vi "Main.vi"(11 "Module Admin":refnum<class "Delacor_lib_QMH_Module Admin.lvclass">) -> ()   [LabVIEW 2022 SP3, in "ActorModule.lvlib"]
doc: "This template is based off of the Queued Message Handler design pattern and the Queued Message Handler project template that ships with LabVIEW.\n\nThe main difference is that the queue is private to this module and communication between modules is performed via Broadcast and Request events.\n\nRequest events are wrapped in public API methods and are handled in the Event Handling Loop (EHL) of this VI. Any module can register for Broadcast events sent by this module. The EHL generates messages based on user interface actions.\n\nThe Message Handling Loop (MHL) processes messages generated by the EHL, or by other messages. The messages are string values, so new messages can be added easily to the Message Cases case structure in the MHL. Each message cluster can also provide an optional value for Message Data, which is a variant that can be converted to whatever message-specific data is required.\n____\nHAMPEL SOFTWARE ENGINEERING v2.6.0 (2023-12-19 10:54)"
uses:
  ActorModule.lvlib
  <vilib>/Delacor/Delacor QMH/Libraries/Module Admin_class/Delacor_lib_QMH_Module Admin.lvclass
  Libraries/hse-libraries/Source/hse-dqmh/Controls/System Message Source.ctl
  Framework/UI Manager/System Message Argument--cluster.ctl
  Module Data--cluster.ctl
  Stop Argument--cluster.ctl
  <vilib>/Delacor/Delacor QMH/Libraries/Message Queue_class/Delacor_lib_QMH_Message Queue.lvclass/Delacor_lib_QMH_Message Queue.ctl
  <vilib>/Delacor/Delacor QMH/Libraries/Module Admin_class/Delacor_lib_QMH_Module Admin.lvclass/Delacor_lib_QMH_Module Admin.ctl
  Prepare Argument--cluster.ctl
  Configure Argument--cluster.ctl
  Request UI Display Argument--cluster.ctl
  Libraries/hse-libraries/Source/hse-dqmh/Controls/Module Display Scenarios.ctl
  Request UI Display (Reply Payload)--cluster.ctl
  Framework/Navigation/Sub-VIs/Ctl Target.ctl
  <vilib>/Utility/miscctls.llb/LVPointTypeDef.ctl
  <vilib>/Delacor/Delacor QMH/Libraries/Message Queue_class/Delacor_lib_QMH_Enqueue Message (Single).vi
  <vilib>/Delacor/Delacor QMH/Libraries/Module Admin_class/Delacor_lib_QMH_Get External Launch.vi
  <vilib>/Utility/error.llb/Error Cluster From Error Code.vi
  <vilib>/ErrorRing/Error Ring.xnode
  <vilib>/Delacor/Delacor QMH/Libraries/Message Queue_class/Delacor_lib_QMH_Message Queue.lvclass
  Libraries/hse-libraries/Source/hse-configuration/config-ini/config-ini.lvclass
  Framework/UI Manager/UI Manager.lvlib
  Libraries/hse-libraries/Source/hse-dqmh/hse-dqmh.lvlib
  <vilib>/Hampel Software Engineering/HSE Logger/hse-logger.lvlib
  Framework/Navigation/Navigation.lvlib
panel:
  out "Message Time":timestamp
  out "Payload":variant
  out "Source":T1
  out "Identifier":string
  in  "Timeout [ms]":u32
  out "Timeout Counter":u32
  out "error out":errorcluster
  # "The \"ActorModule\" serves as an example of a module with a helper loop, which comes with two features: \n\n1. The helper loop can be \"enabled\" to run continuously by using the timeout case of its event structure. It \nwill then increase the timeout counter shown in the indicator below, and it will rotate the selection inside \nthe listbox which is shown in the navigation menu to the left when selecting the \"Actor Module\" button. \n\n2. The helper loop can be registered to receive external events, i.e. broadcasts from other DQMH modules. \nWhen registered for the UI Manager's broadcast event, the indicators below will show any System Message \nthe UI Manager broadcasts, for example whenever a module is removed from the UI Managers subpanel.\n\nThe helper loop can be operated by pressing the \"Actor Module Actions\" button in the navigation menu to \nthe left and then selecting items from the listbox that appears below the button."
  # "Helper Loop - Timeout"
  # "Helper Loop - Broadcast Registration"
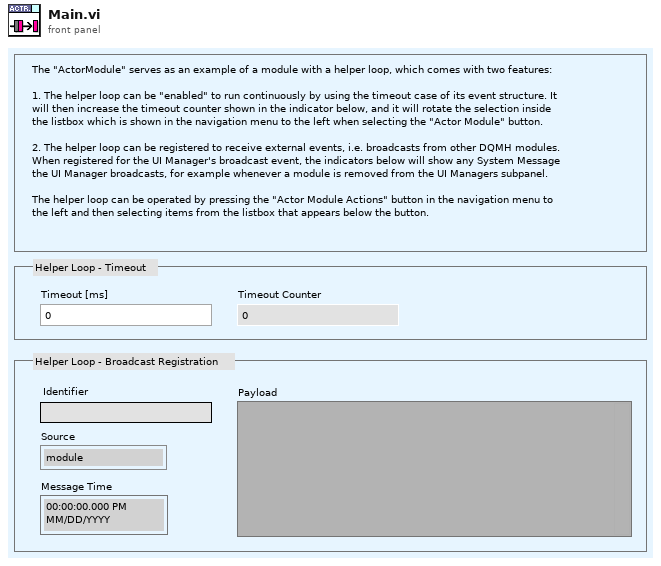
[diagram p1: front panel]
types:
  T1 = typedef "hse-dqmh.lvlib/System Message Source.ctl" = enum16{"module", "application", "network"}
  T2 = typedef "Navigation.lvlib/Broadcast Events--cluster.ctl" = cluster{"Module Did Init":refnum<user-event>, "Status Updated":refnum<user-event>, "Error Reported":refnum<user-event>, "Module Did Stop":refnum<user-event>, "Update Module Execution Status":refnum<user-event>, "Button Pressed":refnum<user-event>, "Sub-Control Pressed":refnum<user-event>, "System Message":refnum<user-event>}
  T3 = typedef "ActorModule.lvlib/Request Events--cluster.ctl" = cluster{"Stop Module":refnum<user-event>, "Show Panel":refnum<user-event>, "Hide Panel":refnum<user-event>, "Get Module Execution Status":refnum<user-event>, "Show Diagram":refnum<user-event>, "Prepare":refnum<user-event>, "Configure":refnum<user-event>, "Enable Actor":refnum<user-event>, "Disable Actor":refnum<user-event>, "Register for System Messages":refnum<user-event>, "Unregister from System Messages":refnum<user-event>, "Request UI Display":refnum<user-event>}
  T4 = typedef "ActorModule.lvlib/Module Data--cluster.ctl" = cluster{"Status":string, "WES Raw Data":cluster{"pdoX":waveform(dbl), "pdoZ":waveform(dbl)}}
  T5 = typedef "Navigation.lvlib/Ctl Target.ctl" = enum16{"Top Button", "Sub ListBox"}
  T6 = enum32{"invalid lock state", "Not Locked", "Locked (No Password)", "Password-protected"}
  T7 = typedef "ActorModule.lvlib/Stop Argument--cluster.ctl" = cluster{"Origin":string, "Exit via Stop Module Req?":bool, "Wait for Module to stop?":bool}
  T8 = typedef "ActorModule.lvlib/Prepare Argument--cluster.ctl" = cluster{"Boolean":bool}
  T9 = typedef "ActorModule.lvlib/Configure Argument--cluster.ctl" = cluster{"Boolean":bool}
  T10 = typedef "ActorModule.lvlib/Request UI Display Argument--cluster.ctl" = cluster{"Scenario":T11, "Wait Notifier":refnum<notifier>, "wait for reply":bool}
  T11 = typedef "hse-dqmh.lvlib/Module Display Scenarios.ctl" = enum16{"Stand-Alone", "Managed"}
  T12 = typedef "LVPointTypeDef.ctl" = cluster{"Horizontal":i16, "Vertical":i16}
  T13 = enum32{"Invalid", "Standard", "Closed", "Hidden", "Minimized", "Maximized"}
  T14 = typedef "ActorModule.lvlib/Request UI Display (Reply Payload)--cluster.ctl" = cluster{"Accept?":bool, "error":errorcluster}
  T15 = typedef "eventsource.ctl" = u32
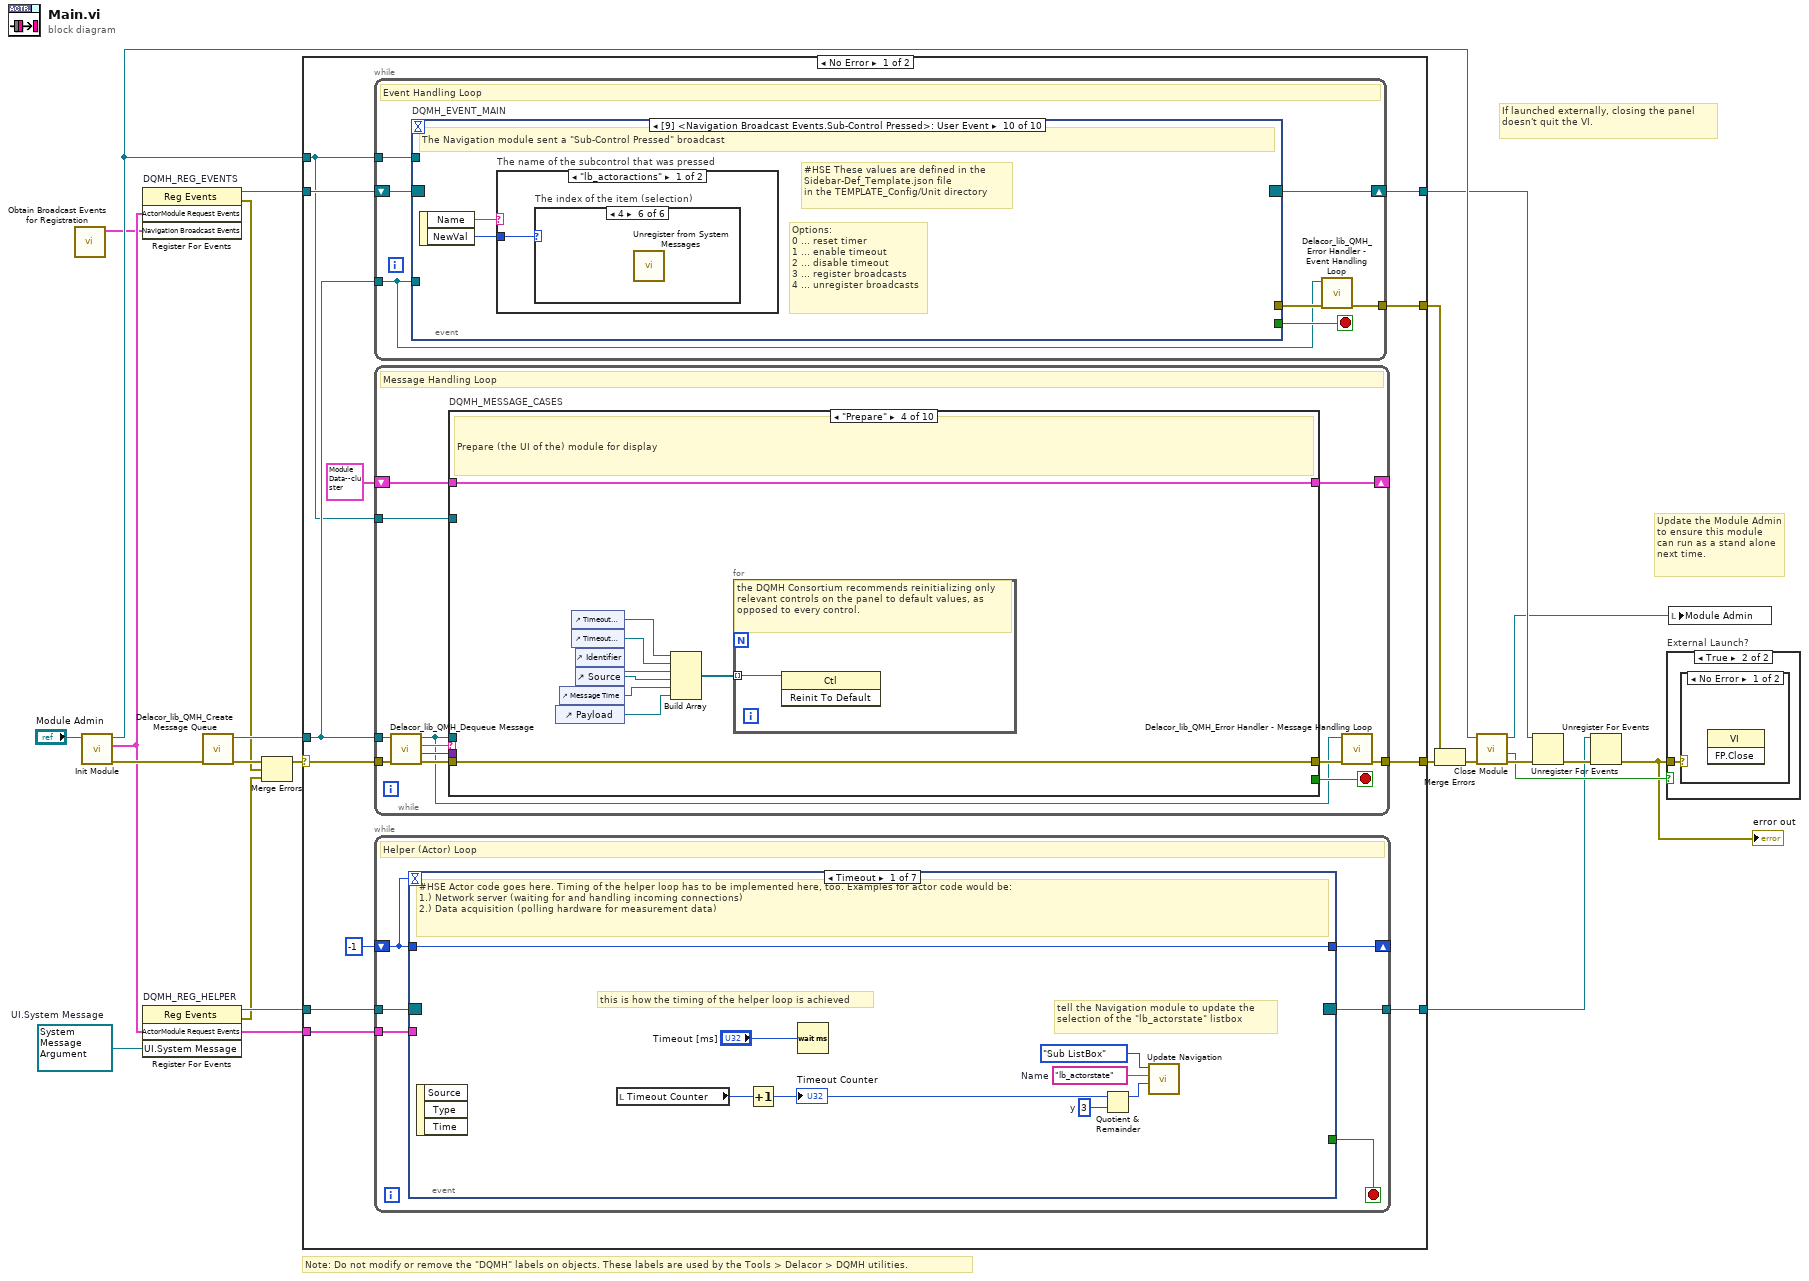
[diagram p0: block diagram]
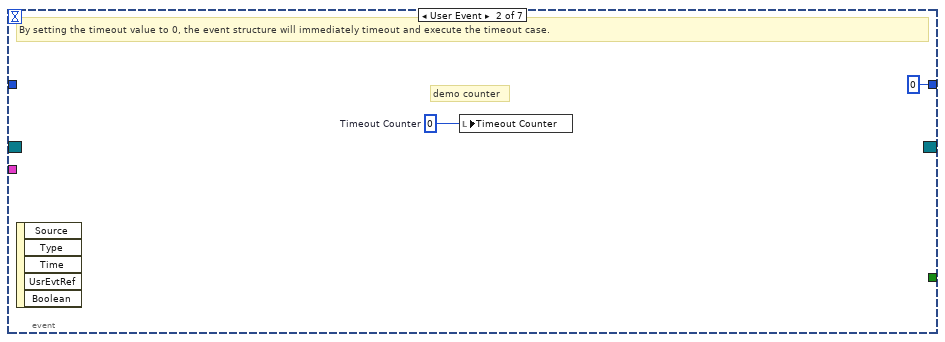
[diagram p2: hidden frame]
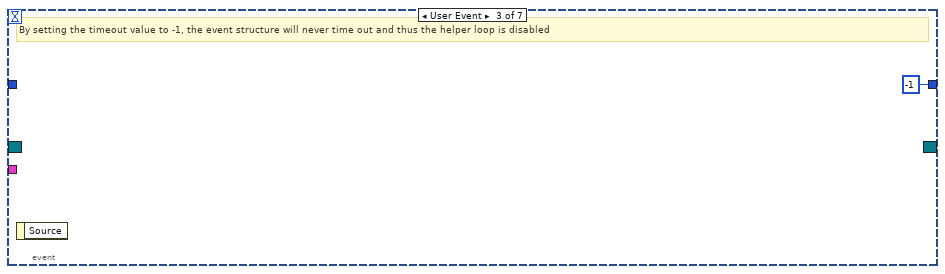
[diagram p3: hidden frame]
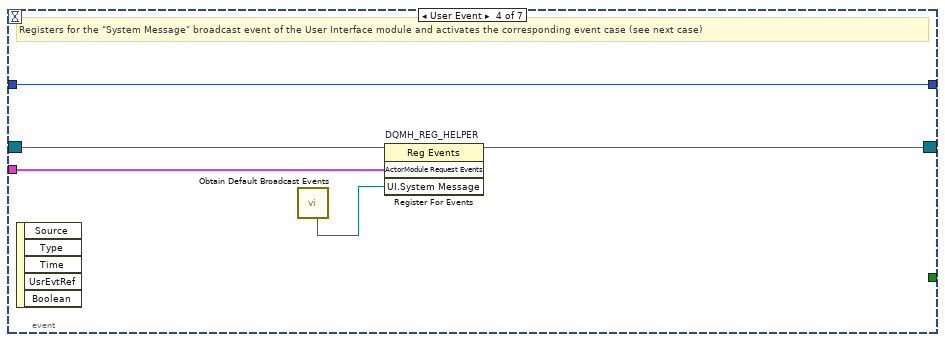
[diagram p4: hidden frame]
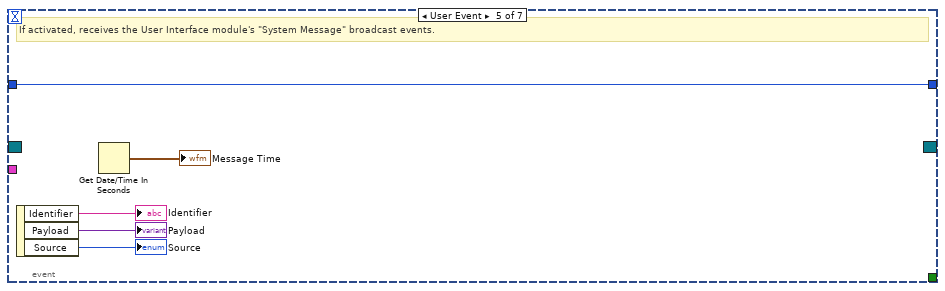
[diagram p5: hidden frame]
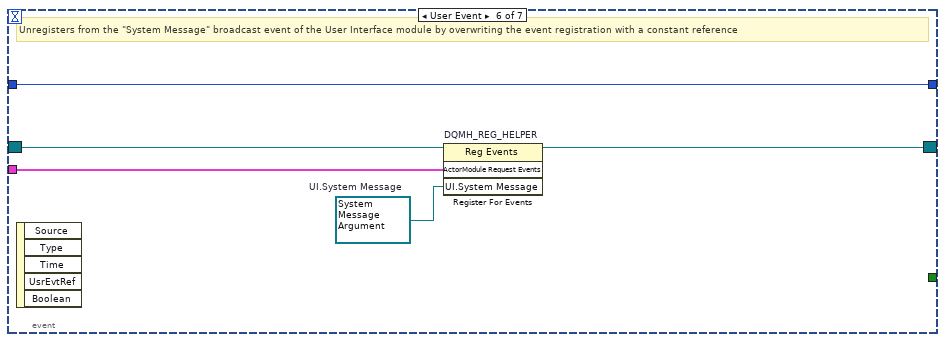
[diagram p6: hidden frame]
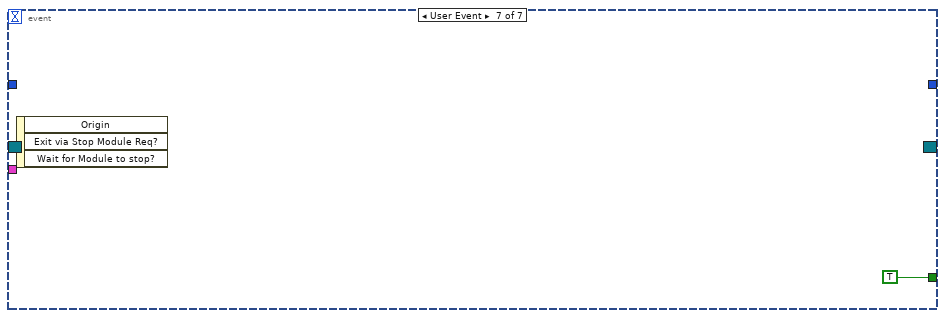
[diagram p7: hidden frame]
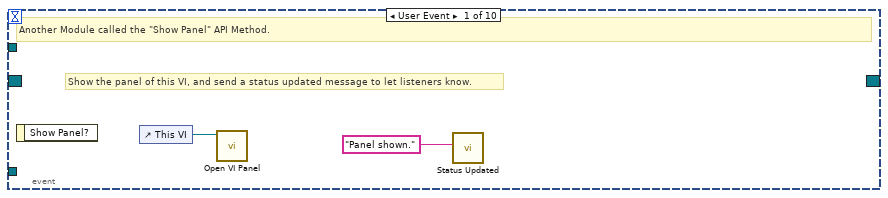
[diagram p8: hidden frame]
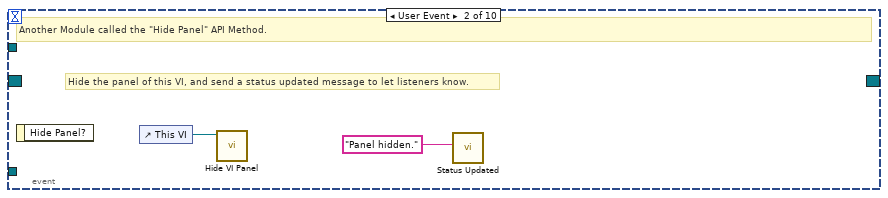
[diagram p9: hidden frame]
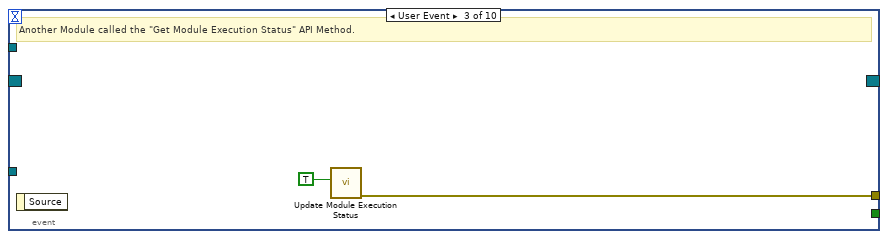
[diagram p10: hidden frame]
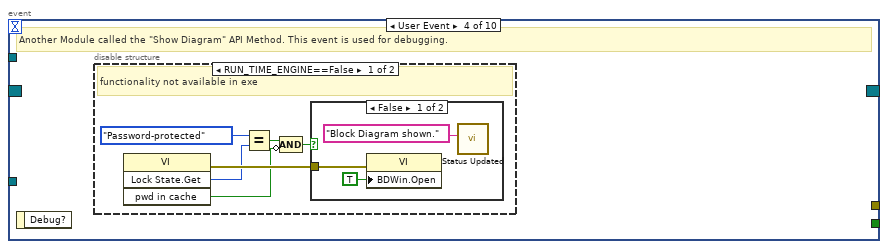
[diagram p11: hidden frame]
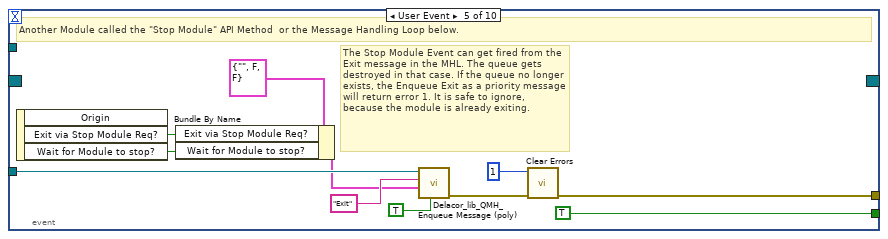
[diagram p14: hidden frame]
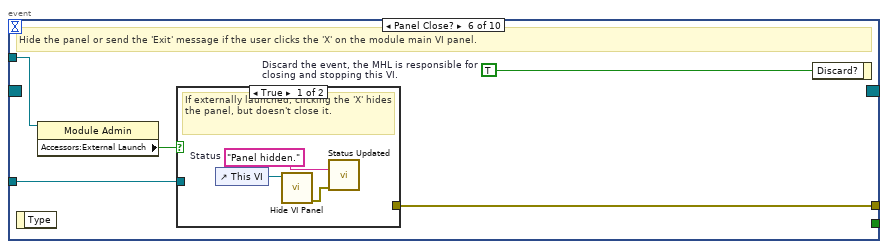
[diagram p15: hidden frame]
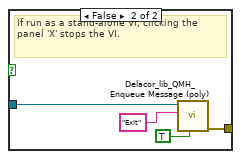
[diagram p16: hidden frame]
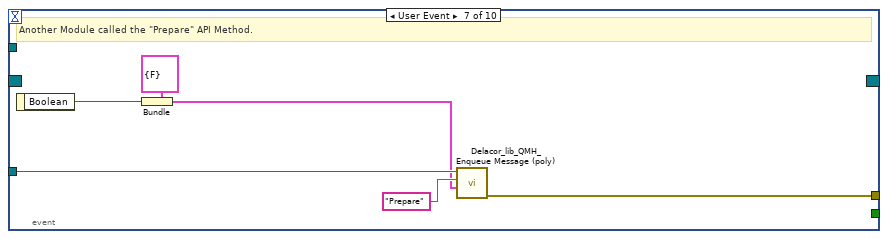
[diagram p17: hidden frame]
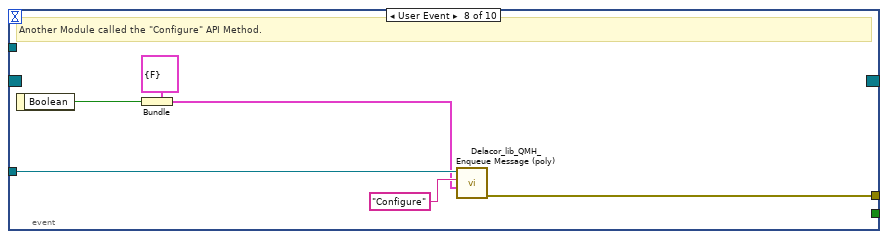
[diagram p18: hidden frame]
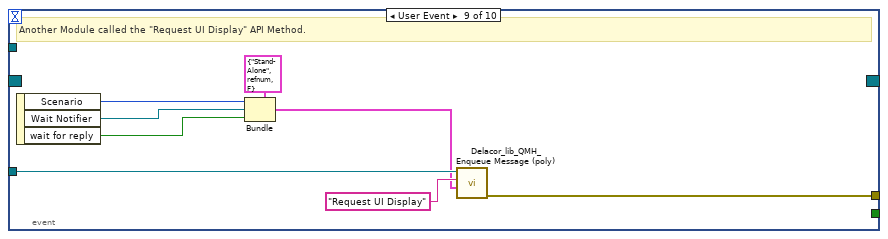
[diagram p19: hidden frame]
diagram:
  w6 = refnum<user-event> refnum  # UI.System Message
  # "If launched externally, closing the panel doesn't quit the VI."
  # "Note: Do not modify or remove the \"DQMH\" labels on objects. These labels are used by the Tools > Delacor > DQMH utilities."
  # "Update the Module Admin to ensure this module can run as a stand alone next time."
  n1 = call "Obtain Broadcast Events for Registration.vi"() -> ("Navigation Broadcast Events"=w1:T2)  [unwired: 9 in, 2 out]
  n2 = call "Init Module.vi"("Singleton Module Admin in"="Module Admin") -> ("error out"=w21:errorcluster, "ActorModule Request Events"=w5:T3, "Singleton Module Admin out"=w23:refnum<class "Delacor_lib_QMH_Module Admin.lvclass">)  [unwired: 8 in]
  n3 = register-events "DQMH_REG_EVENTS"(w5, w1) -> (reference out=w19:refnum<event-registration>, error out=w9:errorcluster)  [unwired: 2 in]
  n4 = register-events "DQMH_REG_HELPER"(w5, w6) -> (reference out=w8:refnum<event-registration>, error out=w7:errorcluster)  [unwired: 2 in]
  n5 = call <vilib>:"Delacor_lib_QMH_Create Message Queue.vi"("error in"=w21) -> ("error out"=w11:errorcluster, "Message Queue"=w18:refnum<class "Delacor_lib_QMH_Message Queue.lvclass">)  [unwired: 9 in]
  n6 = Merge Errors(w11, w9, w7) -> (w10:errorcluster)
  n7 = case shown="No Error" w10 {
    selector: w10 -> [w29 w277]
    tunnel: [w35 w277] -> w22
    tunnel: [w34 w282] -> w20
    tunnel: w19 -> [w32 w282]
    tunnel: w18 -> [w31 w273]
    tunnel: [w30 _] -> w14
    tunnel: w23 -> [w28 w278]
    tunnel: w8 -> [w27 w274]
    tunnel: w5 -> [w25 _]
    tunnel: [w24 w274] -> w2
    frame No Error {
      n8 = while {
        tunnel: w31 -> [w69]
        shift-right: [w74] -> w34
        shift-left: w32 -> [w75]
        tunnel: [w71] -> w30
        tunnel: w28 -> [w70]
        stop <- w72 stop-if-true
        # "Event Handling Loop"
        n9 = event "DQMH_EVENT_MAIN" shown="[9] <Navigation Broadcast Events.Sub-Control Pressed>: User Event" {
          selector: w75 -> [_ _ _ _ _ _ _ _ _ _]
          dyn-events: [_ _ _ _ _ _ _ _ _ _] -> w74
          timeout: _ -> [_ _ _ _ _ _ _ _ _ _]
          tunnel: [_ _ _ _ TRUE ("Discard?") _ _ _ _ _] -> w72
          tunnel: w69 -> [_ _ _ _ w99 w105 w119 w125 w133 _]
          tunnel: [_ _ w81 _ w95 w104 w114 w120 w129 _] -> w73
          tunnel: w70 -> [_ _ _ _ _ w103 _ _ _ _]
          event User Event {
            # "Show the panel of this VI, and send a status updated message to let listeners know."
            # "Another Module called the \"Show Panel\" API Method."
            n10 = event-data() -> ()  [unwired: 1 in, 1 out]
            n11 = control-ref of="This VI"() -> (w77:refnum<vi>)
            n12 = call "Open VI Panel.vi"("VI"=w77) -> ()  [unwired: 10 in, 1 out]
            n13 = call "Status Updated.vi"("Status"="Panel shown." ("format string")) -> ()  [unwired: 10 in, 1 out]
          }
          event User Event {
            # "Hide the panel of this VI, and send a status updated message to let listeners know."
            # "Another Module called the \"Hide Panel\" API Method."
            n14 = event-data() -> ()  [unwired: 1 in, 1 out]
            n15 = control-ref of="This VI"() -> (w79:refnum<vi>)
            n16 = call "Hide VI Panel.vi"("VI"=w79) -> ()  [unwired: 10 in, 1 out]
            n17 = call "Status Updated.vi"("Status"="Panel hidden." ("format string")) -> ()  [unwired: 10 in, 1 out]
          }
          event User Event {
            # "Another Module called the \"Get Module Execution Status\" API Method."
            n18 = event-data() -> ()  [unwired: 1 in, 1 out]
            n19 = call "Update Module Execution Status.vi"("Running?"=TRUE) -> ("error out"=w81:errorcluster)  [unwired: 10 in]
          }
          event User Event {
            # "Another Module called the \"Show Diagram\" API Method. This event is used for debugging."
            n20 = event-data() -> ()  [unwired: 1 in, 1 out]
            n21 = disable-structure shown="RUN_TIME_ENGINE==False" {
              frame condition #0 (active) {
                # "functionality not available in exe"
                n22 = invoke class="VI" method="Lock State.Get"() -> (error out=w87:errorcluster, "Get Lock State"=w86:T6, "pwd in cache"=w83:bool)  [unwired: 4 in, 1 out]
                n23 = Equal?(x=T6."Password-protected", y=w86) -> (x = y?=w84:bool)
                n24 = Compound Arithmetic op=AND(w84, invert w83) -> (w82:bool)
                n25 = case shown="False" w82 {
                  tunnel: w87 -> [w88 _]
                  frame False {
                    n26 = property class="VI"(error in=w88, "BDWin.Open"=TRUE ("Block Diagram Window:Open")) -> ()  [unwired: 1 in, 2 out]
                    n27 = call "Status Updated.vi"("Status"="Block Diagram shown." ("format string")) -> ()  [unwired: 10 in, 1 out]
                  }
                  frame True {
                    # "Password-protected VI, and the password is not in the cache. Do not show the diagram."
                  }
                }
              }
              frame condition #1 {
              }
            }
          }
          event User Event {
            # "The Stop Module Event can get fired from the Exit message in the MHL. The queue gets destroyed in that case. If the queue no longer exists, the Enqueue Exit as a priority message will return error 1. It is safe to ignore, because the module is already exiting."
            # "Another Module called the \"Stop Module\" API Method  or the Message Handling Loop below."
            n28 = event-data() -> ("Exit via Stop Module Req?"=w93:bool, "Wait for Module to stop?"=w92:bool)  [unwired: 1 in, 1 out]
            n29 = Bundle By Name(cluster=T7 {"Origin"="", "Exit via Stop Module Req?"=FALSE, "Wait for Module to stop?"=FALSE} ("Stop Argument"), "Exit via Stop Module Req?"=w93, "Wait for Module to stop?"=w92) -> (w91:T7)
            n30 = call-poly <vilib>:"Delacor_lib_QMH_Enqueue Message (poly).vi"("Priority Message? (F)"=TRUE, "Message Data"=w91, "Message"="Exit", "Message Queue in"=w99) -> ("error out"=w96:errorcluster)  [unwired: 6 in, 1 out]
            n31 = call <vilib>:"Clear Errors.vi"("error in (no error)"=w96, "specific error code to clear (0: all)"=1) -> ("error out"=w95:errorcluster)  [unwired: 4 in, 1 out]
          }
          event Panel Close? {
            w106 = TRUE  # Discard the event, the MHL is responsible for closing and stopping this VI.
            # "Hide the panel or send the 'Exit' message if the user clicks the 'X' on the module main VI panel."
            n32 = event-data() -> ()  [unwired: 1 in, 1 out]
            n33 = property class="Module Admin"(reference=w103) -> ("Accessors:External Launch"=w102:bool)  [unwired: 1 in, 2 out]
            n34 = case shown="True" w102 {
              tunnel: w105 -> [_ w113]
              tunnel: [_ w112] -> w104
              frame True {
                w108 = "Panel hidden."  # Status
                # "If externally launched, clicking the 'X' hides the panel, but doesn't close it."
                n35 = control-ref of="This VI"() -> (w109:refnum<vi>)
                n36 = call "Hide VI Panel.vi"("VI"=w109) -> ("error out"=w107:errorcluster)  [unwired: 10 in]
                n37 = call "Status Updated.vi"("error in (no error)"=w107, "Status"=w108) -> ()  [unwired: 9 in, 1 out]
              }
              frame False {
                # "If run as a stand-alone VI, clicking the panel 'X' stops the VI."
                n38 = call-poly <vilib>:"Delacor_lib_QMH_Enqueue Message (poly).vi"("Priority Message? (F)"=TRUE, "Message"="Exit", "Message Queue in"=w113) -> ("error out"=w112:errorcluster)  [unwired: 7 in, 1 out]
              }
            }
            n39 = event-data("Discard?"=w106) -> ()  [unwired: 1 in, 1 out]
          }
          event User Event {
            # "Another Module called the \"Prepare\" API Method."
            n40 = event-data() -> ("Boolean"=w115:bool)  [unwired: 1 in]
            n41 = Bundle(cluster=T8 {"Boolean"=FALSE} ("Prepare Argument"), "Boolean"=w115) -> (w116:T8)
            n42 = call-poly <vilib>:"Delacor_lib_QMH_Enqueue Message (poly).vi"("Message Data"=w116, "Message"="Prepare", "Message Queue in"=w119) -> ("error out"=w114:errorcluster)  [unwired: 7 in, 1 out]
          }
          event User Event {
            # "Another Module called the \"Configure\" API Method."
            n43 = event-data() -> ("Boolean"=w121:bool)  [unwired: 1 in]
            n44 = Bundle(cluster=T9 {"Boolean"=FALSE} ("Configure Argument"), "Boolean"=w121) -> (w122:T9)
            n45 = call-poly <vilib>:"Delacor_lib_QMH_Enqueue Message (poly).vi"("Message Data"=w122, "Message"="Configure", "Message Queue in"=w125) -> ("error out"=w120:errorcluster)  [unwired: 7 in, 1 out]
          }
          event User Event {
            # "Another Module called the \"Request UI Display\" API Method."
            n46 = event-data() -> ("Scenario"=w128:T11, "Wait Notifier"=w127:refnum<notifier>, "wait for reply"=w126:bool)  [unwired: 1 in]
            n47 = Bundle(cluster=T10 {"Scenario"=enum."Stand-Alone", "Wait Notifier"=refnum, "wait for reply"=FALSE} ("Display Module UI Argument"), "Scenario"=w128, "Wait Notifier"=w127, "wait for reply"=w126) -> (w130:T10)
            n48 = call-poly <vilib>:"Delacor_lib_QMH_Enqueue Message (poly).vi"("Message Data"=w130, "Message"="Request UI Display", "Message Queue in"=w133) -> ("error out"=w129:errorcluster)  [unwired: 7 in, 1 out]
          }
          event User Event {
            # "#HSE These values are defined in the\nSidebar-Def_Template.json file \nin the TEMPLATE_Config/Unit directory"
            # "Options:\n0 ... reset timer\n1 ... enable timeout\n2 ... disable timeout\n3 ... register broadcasts\n4 ... unregister broadcasts"
            # "The Navigation module sent a \"Sub-Control Pressed\" broadcast"
            n49 = event-data() -> ("Name"=w135:string, "NewVal"=w134:i32)  [unwired: 1 in]
            n50 = case "The name of the subcontrol that was pressed" shown="\"lb_actoractions\"" w135 {
              tunnel: w134 -> [w136 _]
              frame "lb_actoractions" {
                n51 = case "The index of the item (selection)" shown="4" w136 {
                  frame Default {
                  }
                  frame 0 {
                    n52 = local write "Timeout [ms]"(u32 1000 ("Timeout Wait [ms]")) -> ()
                  }
                  frame 1 {
                    n53 = call "Enable Actor.vi"() -> ()  [unwired: 11 in, 1 out]
                  }
                  frame 2 {
                    n54 = call "Disable Actor.vi"() -> ()  [unwired: 11 in, 1 out]
                  }
                  frame 3 {
                    n55 = call "Register for System Messages.vi"() -> ()  [unwired: 11 in, 1 out]
                  }
                  frame 4 {
                    n56 = call "Unregister from System Messages.vi"() -> ()  [unwired: 11 in, 1 out]
                  }
                }
              }
              frame Default {
              }
            }
          }
        }
        n57 = call-dynamic "Delacor_lib_QMH_Error Handler - Event Handling Loop.vi"("error in"=w73, "Message Queue in"=w69) -> ("dup error in"=w71:errorcluster)  [unwired: 8 in, 1 out]
      }
      n58 = while {
        tunnel: w31 -> [w141]
        shift-right: [w147] -> _
        shift-left: T4 {"Status"="", "WES Raw Data"={"pdoX"={"t0"=timestamp(0 s since 1904-01-01), "dt"=1.0, "Y"=[]}, "pdoZ"={"t0"=timestamp(0 s since 1904-01-01), "dt"=1.0, "Y"=[]}}} ("Data Cluster") -> [w148]
        tunnel: w29 -> [w145]
        tunnel: [w139] -> w35
        tunnel: w28 -> [w138]
        stop <- w146 stop-if-true
        # "Message Handling Loop"
        n59 = call-dynamic "Delacor_lib_QMH_Dequeue Message.vi"("error in"=w145, "Message Queue in"=w141) -> ("error out"=w144:errorcluster, "Message Data"=w142:variant, "Message"=w143:string, "Message Queue out"=w140:refnum<class "Delacor_lib_QMH_Message Queue.lvclass">)  [unwired: 6 in]
        n60 = case "DQMH_MESSAGE_CASES" shown="\"Prepare\"" w143 {
          selector: w143 -> [_ _ _ _ _ _ _ _ _ w262]
          tunnel: w140 -> [_ _ _ _ _ _ _ w233 w256 _]
          tunnel: w144 -> [w157 w169 w176 w197 w211 w225 w227 w239 w258 w259]
          tunnel: [w152 w169 w187 w197 w203 w223 w227 w230 w252 w260] -> w149
          tunnel: w148 -> [w156 w168 w189 w198 w210 w224 w226 w238 w255 w264]
          tunnel: [w156 w168 w189 w198 w210 w224 w226 w238 w255 w264] -> w147
          tunnel: [_ _ _ _ _ _ _ _ w254 _] -> w146
          tunnel: w142 -> [_ _ _ _ w208 _ _ w237 w251 _]
          tunnel: w138 -> [w158 _ _ _ _ _ _ w232 w244 _]
          frame "Initialize" {
            # "Initialize - Any operation that needs to be done before the module can receive messages. Synchronize Caller Events.vi will inform Start Module.vi that the module has launched and is ready to receive messages. Module Did Init.vi will broadcast that the module initialized."
            n61 = call "Synchronize Caller Events.vi"("error in (no error)"=w157, "Singleton Module Admin in"=w158) -> ("error out"=w153:errorcluster, "Singleton Module Admin out"=w151:refnum<class "Delacor_lib_QMH_Module Admin.lvclass">)  [unwired: 8 in]
            n62 = property class="Module Admin"(reference=w151) -> ("Accessors:External Launch"=w162:bool)  [unwired: 1 in, 2 out]
            n63 = property on="Pane" class="Pane"("Origin"=T12 {"Horizontal"=0, "Vertical"=0}) -> ()  [unwired: 2 in, 2 out]
            n64 = Select(t=T13."Hidden" ("State"), s=w162, f=T13."Standard" ("State")) -> (s? t:f=w159:T13)
            n65 = call "Module Name--constant.vi"() -> ("Module Name"=w167:string)  [unwired: 11 in]
            n66 = property class="VI"("Front Panel.Title"=w167) -> (reference out=w165:refnum<vi>, error out=w166:errorcluster)  [unwired: 2 in]
            n67 = call "Module Name--constant.vi"() -> ("Module Name"=w154:string)  [unwired: 11 in]
            n68 = invoke class="VI" method="FP.Open"(reference=w165, error in=w166, "State"=w159) -> (reference out=w164:refnum<vi>, error out=w163:errorcluster)  [unwired: 2 in, 3 out]
            n69 = call "Module Did Init.vi"("error in (no error)"=w153, "Initialized?"=TRUE, "Origin"=w154) -> ("error out"=w152:errorcluster)  [unwired: 8 in]
            n70 = invoke class="VI" method="FP.Center"(reference=w164, error in=w163) -> ()  [unwired: 1 in, 3 out]
          }
          frame "--- Module Specific ---" {
            # "Separator -- The following cases handle messages specific to this Module."
          }
          frame "Configure" {
            # "Set the helper loop's timing"
            # "Read a string value from the .ini-file"
            # "<appname> is defined in /Project/PROJECT_Name.vi\n<unit-id> is defined in <appname>_Config/config.ini\n<modulename> is the name of this module"
            # "Open the module-specific configuration file, which can be found in\n<appname>_Config/Unit_<unit-id>/<modulename>.ini"
            # "Triggers the auto-configuration of the module"
            n71 = call "Module Name--constant.vi"() -> ("Module Name"=w177:string)  [unwired: 11 in]
            n72 = call "Create Module Config.vi"("error in"=w176, "DQMH Module Name"=w177) -> ("error out"=w175:errorcluster, "config-ini out"=w174:refnum<class "config-ini.lvclass">)  [unwired: 8 in]
            n73 = control-ref of="This VI"() -> (w178:refnum<vi>)
            n74 = call-dynamic "Read String.vi"("Section"="global", "error in"=w175, "Key"="descriptor", "config-base in"=w174) -> ("error out"=w181:errorcluster, "Value"=w179:string, "config-base out"=w180:refnum<class "config-ini.lvclass">)  [unwired: 5 in]
            n75 = call "DQMH System Message - Add to Run-Time Menu.vi"("Module Descriptor"=w179, "Main VI Reference"=w178) -> ("Payload"=w183:variant, "Identifier"=w184:string, "Source"=w185:T1)  [unwired: 7 in]
            n76 = property class="VI"("Front Panel.Title"=w179) -> ()  [unwired: 2 in, 2 out]
            n77 = call "System Message.vi"("Sys. Msg. Source"=w185, "Payload"=w183, "Identifier"=w184) -> ()  [unwired: 8 in, 1 out]
            n78 = call-dynamic "Read String.vi"("Section"="section-name", "error in"=w181, "Key"="key-name", "config-base in"=w180) -> ("error out"=w188:errorcluster)  [unwired: 5 in, 2 out]
            n79 = local write "Timeout [ms]"(u32 500 ("Timeout Wait [ms]")) -> ()
            n80 = call <vilib>:"INFO.vi"("Message"="Module User Interface configured.", "error in"=w188) -> ("error out"=w187:errorcluster)  [unwired: 9 in]
          }
          frame "Prepare" {
            # "Prepare (the UI of the) module for display"
            n81 = control-ref of="Payload"() -> (w191:refnum<vi>)
            n82 = control-ref of="Message Time"() -> (w192:refnum<vi>)
            n83 = control-ref of="Timeout [ms]"() -> (w196:refnum<vi>)
            n84 = control-ref of="Timeout Counter"() -> (w195:refnum<vi>)
            n85 = control-ref of="Identifier"() -> (w194:refnum<vi>)
            n86 = control-ref of="Source"() -> (w193:refnum<vi>)
            n87 = Build Array(w196, w195, w194, w193, w192, w191) -> (w190:refnum<vi>[])
            n88 = for {
              tunnel: w190 -> [w199] mode=indexing
              # "the DQMH Consortium recommends reinitializing only relevant controls on the panel to default values, as opposed to every control."
              n89 = invoke class="Ctl" method="Reinit To Default"(reference=w199) -> ()  [unwired: 2 in, 3 out]
            }
          }
          frame "Request UI Display" {
            # "Requests the module to display its UI as specified in <b>Scenario</b>:\n\"managed\" => in the UI Manager's subpanel\n\"stand-alone\" => as a separate window"
            n90 = Variant To Data(error in=w211, type=T10 {"Scenario"=enum."Stand-Alone", "Wait Notifier"=refnum, "wait for reply"=FALSE} ("Request UI Display Argument"), Variant=w208) -> (data=w206:T10, error out=w209:errorcluster)
            n91 = Unbundle By Name(w206) -> ("Scenario"=w202:T11, "Wait Notifier"=w205:refnum<notifier>, "wait for reply"=w204:bool)
            n92 = control-ref of="This VI"() -> (w201:refnum<vi>)
            n93 = case shown="\"Managed\"" w202 {
              tunnel: w201 -> [w213 w218]
              tunnel: [w212 w214] -> w200
              frame "Stand-Alone", Default {
                n94 = call "Open VI Panel.vi"("VI"=w213) -> ("error out"=w212:errorcluster)  [unwired: 10 in]
              }
              frame "Managed" {
                n95 = call "DQMH System Message - Ready for Display.vi"("Main VI Reference"=w218) -> ("Payload"=w215:variant, "Identifier"=w216:string, "Source"=w217:T1)  [unwired: 8 in]
                n96 = call "System Message.vi"("Sys. Msg. Source"=w217, "Payload"=w215, "Identifier"=w216) -> ("error out"=w214:errorcluster)  [unwired: 8 in]
              }
            }
            n97 = Merge Errors(w209, w200) -> (w203:errorcluster)
            n98 = case shown="True" w204 {
              tunnel: w205 -> [_ w222]
              tunnel: w200 -> [_ w221]
              frame False {
              }
              frame True {
                n99 = Bundle By Name(cluster=T14 {"Accept?"=FALSE, "error"={"status"=FALSE, "code"=0, "source"=""}} ("Request UI Display (Reply Payload)"), "error"=w221) -> (w219:T14)
                n100 = Send Notification(notification=w219, notifier=w222) -> ()  [unwired: 1 in, 2 out]
              }
            }
          }
          frame "---Copy This Frame---" {
            # "Duplicate this frame when creating new messages.  Change this comment in the duplicated frame to describe this message."
            n101 = Merge Errors(w225) -> (w223:errorcluster)
          }
          frame "--- Exit and Error Handling---" {
            # "Separator - The following cases handle errors and exit messages."
          }
          frame "Error" {
            # "Error - Check the error message data and respond accordingly. This message is sent by the \"Error Handler\" VIs at the end of each loop in this application."
            n102 = property class="Module Admin"(reference=w232) -> ("Accessors:External Launch"=w231:bool)  [unwired: 1 in, 2 out]
            n103 = Variant To Data(error in=w239, type=errorcluster {"status"=FALSE, "code"=0, "source"=""} ("error constant"), Variant=w237) -> (data=w229:errorcluster, error out=w235:errorcluster)
            n104 = call "Error Reported.vi"("Error"=w229) -> ()  [unwired: 10 in, 1 out]
            n105 = call <vilib>:"ERROR.vi"("Message"="DQMH Error Case", "error in"=w229) -> ()  [unwired: 9 in, 1 out]
            n106 = case shown="False" w231 {
              tunnel: [w243 _] -> w234
              tunnel: w233 -> [w242 _]
              tunnel: w229 -> [_ _]
              frame False {
                # "If the module is running standalone, then pop up an error dialog and call the \"Exit\" message."
                n107 = call-poly <vilib>:"Delacor_lib_QMH_Enqueue Message (poly).vi"("Priority Message? (F)"=TRUE, "Message"="Exit", "Message Queue in"=w242) -> ("error out"=w243:errorcluster)  [unwired: 7 in, 1 out]
              }
              frame True {
                # "If the module was launched externally, calling the Error Reported broadcast VI is the only action performed by the \"Error\" message. The module's caller can then process the error appropriately."
              }
            }
            n108 = Merge Errors(w235, w234) -> (w230:errorcluster)
            n109 = local write "error out"(w230) -> ()
          }
          frame "Exit" {
            w249 = 91  # 91: not all Exit messages will have an argument
            w254 = TRUE  # Stop the VI
            # "Release the message queue reference"
            # "#CodeNeeded - Add any required cleanup code here"
            # "Exit - Exit the application."
            n110 = Variant To Data(error in=w258, type=T7 {"Origin"="", "Exit via Stop Module Req?"=FALSE, "Wait for Module to stop?"=FALSE} ("Stop Argument"), Variant=w251) -> (data=w247:T7, error out=w250:errorcluster)
            n111 = call <vilib>:"Clear Errors.vi"("error in (no error)"=w250, "specific error code to clear (0: all)"=w249) -> ("error out"=w257:errorcluster)  [unwired: 4 in, 1 out]
            n112 = control-ref of="This VI"() -> (w245:refnum<vi>)
            n113 = call-dynamic "Delacor_lib_QMH_Release Message Queue.vi"("error in"=w257, "Message Queue"=w256) -> ("error out"=w253:errorcluster)  [unwired: 9 in]
            n114 = call "Handle Exit.vi"("Stop Argument"=w247, "Admin in"=w244, "VI reference"=w245) -> ("error out"=w246:errorcluster)  [unwired: 7 in, 1 out]
            n115 = Merge Errors(w253, w246) -> (w252:errorcluster)
            n116 = call "Error Reported.vi"("Error"=w252) -> ()  [unwired: 10 in, 1 out]
          }
          frame Default {
            # "'Default' case only runs if there is a message that isn't defined in any of the other cases.  Output a programming error."
            n117 = call "Module Name--constant.vi"() -> ("Module Name"=w261:string)  [unwired: 11 in]
            n118 = xnode "Error Ring"("parameter 0"=w262, "parameter 1"=w261) -> ("error out"=w263:errorcluster)
            n119 = Merge Errors(w259, w263) -> (w260:errorcluster)
          }
        }
        n120 = call-dynamic "Delacor_lib_QMH_Error Handler - Message Handling Loop.vi"("error in"=w149, "Message Queue in"=w140) -> ("dup error in"=w139:errorcluster)  [unwired: 8 in, 1 out]
      }
      n121 = while "DQMH_HELPER_LOOP" {
        tunnel: w27 -> [w41]
        shift-right: [w38] -> _
        shift-left: -1 -> [w39]
        tunnel: w25 -> [w37]
        tunnel: [w36] -> w24
        stop <- w40 stop-if-true
        # "Helper (Actor) Loop"
        n122 = event shown="[0] Timeout" {
          selector: w41 -> [_ _ _ w56 _ w64 _]
          dyn-events: [_ _ _ w55 _ w63 _] -> w36
          timeout: w39 -> [_ _ _ _ _ _ _]
          tunnel: [_ _ _ _ _ _ TRUE] -> w40
          tunnel: [w49 0 -1 w57 w62 w67 _] -> w38
          tunnel: w39 -> [w49 _ _ w57 w62 w67 _]
          tunnel: w37 -> [_ _ _ w54 _ w65 _]
          event Timeout {
            w43 = u32 3  # y
            w45 = "lb_actorstate"  # Name
            # "this is how the timing of the helper loop is achieved"
            # "tell the Navigation module to update the selection of the \"lb_actorstate\" listbox"
            # "#HSE Actor code goes here. Timing of the helper loop has to be implemented here, too. Examples for actor code would be:\n1.) Network server (waiting for and handling incoming connections)\n2.) Data acquisition (polling hardware for measurement data)"
            n123 = event-data() -> ()  [unwired: 1 in, 3 out]
            n124 = local read "Timeout Counter"() -> (w48:u32)
            n125 = Increment(x=w48) -> (x+1=w44:u32)
            "Timeout Counter" <- w44
            n126 = Wait (ms)(milliseconds to wait="Timeout [ms]") -> ()  [unwired: 1 out]
            n127 = Quotient & Remainder(x=w44, y=w43) -> (x-y*floor(x/y)=w42:u32)  [unwired: 1 out]
            n128 = call "Update Navigation.vi"("Data"=w42, "Name"=w45, "Ctl Target"=Ctl_Target."Sub ListBox") -> ()  [unwired: 8 in, 1 out]
          }
          event User Event {
            w50 = u32 0  # Timeout Counter
            # "demo counter"
            # "By setting the timeout value to 0, the event structure will immediately timeout and execute the timeout case."
            n129 = event-data() -> ()  [unwired: 1 in, 5 out]
            n130 = local write "Timeout Counter"(w50) -> ()
          }
          event User Event {
            # "By setting the timeout value to -1, the event structure will never time out and thus the helper loop is disabled"
            n131 = event-data() -> ()  [unwired: 1 in, 1 out]
          }
          event User Event {
            # "Registers for the \"System Message\" broadcast event of the User Interface module and activates the corresponding event case (see next case)"
            n132 = event-data() -> ()  [unwired: 1 in, 5 out]
            n133 = call "Obtain Default Broadcast Events.vi"() -> ("System Message"=w53:refnum<user-event>)  [unwired: 6 in, 5 out]
            n134 = register-events "DQMH_REG_HELPER"(reference=w56, w54, w53) -> (reference out=w55:refnum<event-registration>)  [unwired: 1 in, 1 out]
          }
          event User Event {
            # "If activated, receives the User Interface module's \"System Message\" broadcast events."
            n135 = event-data() -> ("Identifier"=→"Identifier":string, "Payload"=→"Payload":variant, "Source"=→"Source":T15)  [unwired: 1 in]
            n136 = Get Date/Time In Seconds() -> (seconds since 1Jan1904=→"Message Time":timestamp)
          }
          event User Event {
            w66 = refnum<user-event> refnum  # UI.System Message
            # "Unregisters from the \"System Message\" broadcast event of the User Interface module by overwriting the event registration with a constant reference"
            n137 = event-data() -> ()  [unwired: 1 in, 5 out]
            n138 = register-events "DQMH_REG_HELPER"(reference=w64, w65, w66) -> (reference out=w63:refnum<event-registration>)  [unwired: 1 in, 1 out]
          }
          event User Event {
            n139 = event-data() -> ()  [unwired: 1 in, 3 out]
          }
        }
      }
    }
    frame Error {
      # "Synchronize Caller Events.vi will inform Start Module.vi that the module has launched and will let the code calling Start Module.vi register for broadcasts and would permit the caller receive the broadcast that an error occurred at launch time."
      n140 = call-dynamic "Delacor_lib_QMH_Release Message Queue.vi"("Message Queue"=w273) -> ()  [unwired: 10 in, 1 out]
      n141 = call "Synchronize Caller Events.vi"("Singleton Module Admin in"=w278) -> ("error out"=w275:errorcluster)  [unwired: 9 in, 1 out]
      n142 = call "Module Name--constant.vi"() -> ("Module Name"=w281:string)  [unwired: 11 in]
      n143 = Format Into String(format string="An error occurred during initialization. %s is no longer running.", w281) -> (resulting string=w279:string)  [unwired: 2 in, 1 out]
      n144 = Merge Errors(w277, w275) -> (w276:errorcluster)
      n145 = call "Error Reported.vi"("Additional Information"=w279, "Error"=w276) -> ()  [unwired: 9 in, 1 out]
    }
  }
  n146 = Merge Errors(w14, w22) -> (w13:errorcluster)
  n147 = call "Close Module.vi"("error in (no error)"=w13, "Module Admin in"=w23) -> ("error out"=w16:errorcluster, "External Launch"=w12:bool, "Module Admin out"=w15:refnum<class "Delacor_lib_QMH_Module Admin.lvclass">)  [unwired: 7 in]
  n148 = Unregister For Events(event registration refnum=w20, error in=w16) -> (error out=w4:errorcluster)
  n149 = Unregister For Events(event registration refnum=w2, error in=w4) -> (error out=w3:errorcluster)
  "error out" <- w3
  n150 = case "External Launch?" shown="True" w12 {
    tunnel: w3 -> [_ w283]
    frame False {
    }
    frame True {
      n151 = case shown="No Error" w283 {
        frame No Error {
          n152 = invoke class="VI" method="FP.Close"() -> ()  [unwired: 3 in, 3 out]
        }
        frame Error {
          n153 = invoke class="VI" method="FP.Open"("Activate"=TRUE ("Activate?")) -> ()  [unwired: 4 in, 5 out]
        }
      }
    }
  }
  n154 = local write "Module Admin"(w15) -> ()
